vi "HO5_Generator#2.vi"(3 "?":bool, 4 "Delay (ms)":i16=500, 5 "Min":dbl=100.0, 6 "Max":dbl=500.0) -> (2 "Strip Chart":T2(graph))   [LabVIEW 2020]
panel:
  in  "Averaged Points":i16=5 min=1 max=1024 step=1
  out "Biggest/Smallest value":T1 {"Big time" format="%<%.3X>T"}
  out "Countdown (s)":dbl caption="Elapsed Time (s)"
  in  "Time Target (20)":dbl=20.0
  out "Current Overall average":dbl
  out "When slope is >0, than it's green.":bool
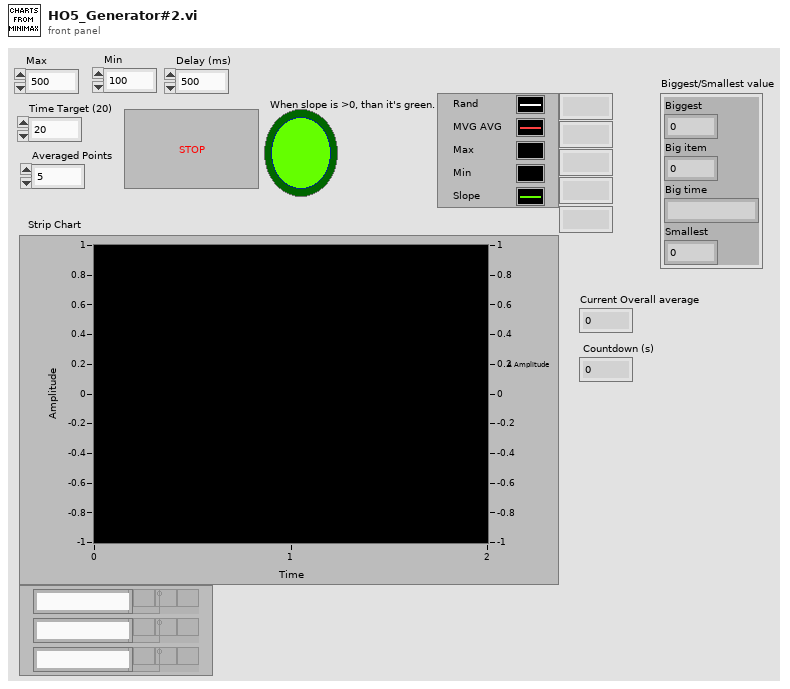
[diagram p1: front panel]
types:
  T1 = cluster{"Biggest":dbl, "Big item":i32, "Big time":timestamp, "Smallest":dbl}
  T2 = cluster{"Double":dbl, dbl, "Max":dbl, "Min":dbl, "Linear Slope":dbl}
  T3 = cluster{"Double":dbl, dbl, "Max":dbl, "Min":dbl, "Linear Slope":dbl}[]
  T4 = cluster{"Double":dbl, dbl, "Max":dbl, "Min":dbl, "Theta (degree)":dbl}
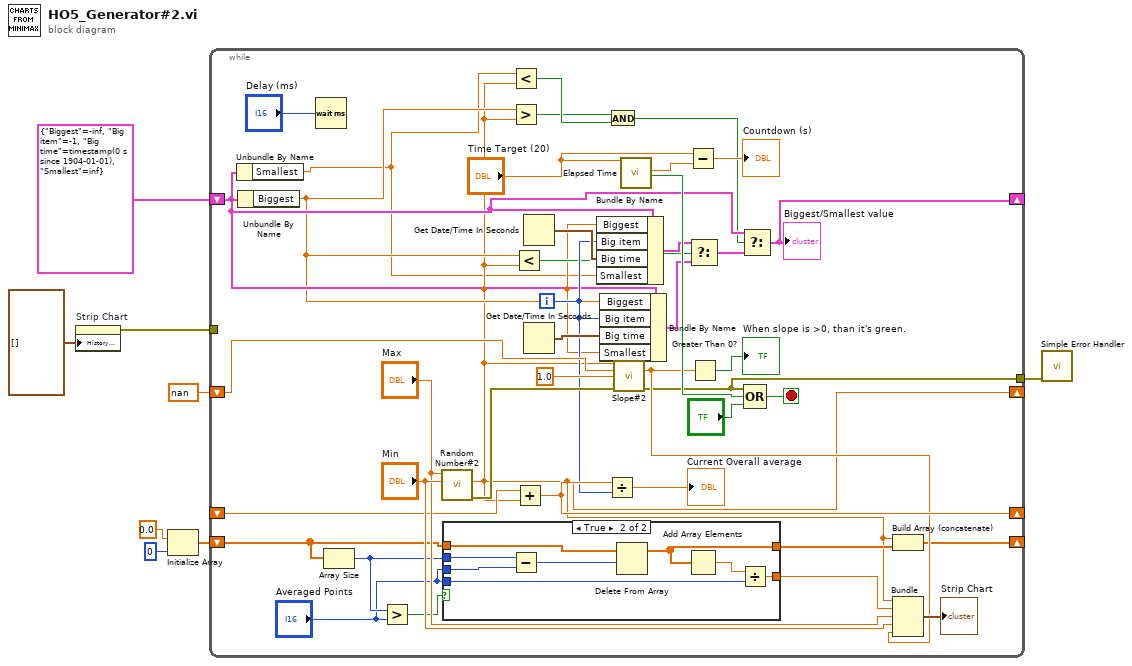
[diagram p0: block diagram]
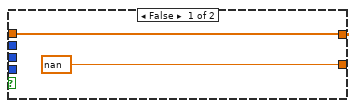
[diagram p2: hidden frame]
diagram:
  n1 = property on="Strip Chart" class="WFChart (strict)"("History Data"=T3 []) -> (error out=w8:errorcluster)  [unwired: 2 in, 1 out]
  n2 = Initialize Array(0.0 ("element"), 0 ("dimension size")) -> (w1:dbl[])
  n3 = while {
    tunnel: w8 -> [_]
    shift-right: [w42] -> _
    shift-left: _ -> [w43]
    tunnel: [w33] -> w6
    shift-right: [w12] -> _
    shift-left: nan -> [w32]
    shift-right: [w30] -> _
    shift-left: T1 {"Biggest"=-inf, "Big item"=-1, "Big time"=timestamp(0 s since 1904-01-01), "Smallest"=inf} -> [w26]
    shift-right: [w20] -> _
    shift-left: w1 -> [w18]
    i -> [w27]
    stop <- w41 stop-if-true
    n4 = Unbundle By Name(w26) -> ("Smallest"=w11:dbl)
    n5 = Unbundle By Name(w26) -> ("Biggest"=w13:dbl)
    n6 = Wait (ms)(milliseconds to wait="Delay (ms)") -> ()  [unwired: 1 out]
    n7 = Array Size(array=w18) -> (size(s)=w17:i32)
    n8 = Greater?(x=w17, y="Averaged Points") -> (0:w19:bool)
    n9 = call "Random Number#2.vi"("Maximum"="Max", "Minimum"="Min") -> ("Double"=w12:dbl, "error out"=w34:errorcluster)  [unwired: 4 in, 2 out]
    n10 = case shown="True" w19 {
      tunnel: w18 -> [w51 w59]
      tunnel: w17 -> [_ w57]
      tunnel: "Averaged Points" -> [_ w56]
      tunnel: "Averaged Points" -> [_ w55]
      tunnel: [nan w54] -> w15
      tunnel: [w51 w52] -> w14
      frame False {
      }
      frame True {
        n11 = Subtract(x=w57, y=w56) -> (x-y=w58:i32)
        n12 = Delete From Array(array=w59, length=w58) -> (array with subset deleted=w52:dbl[])  [unwired: 1 in, 1 out]
        n13 = Add Array Elements(numeric array=w52) -> (sum=w53:dbl)
        n14 = Divide(x=w53, y=w55) -> (x/y=w54:dbl)
      }
    }
    n15 = Less?(x=w11, y=w12) -> (x < y?=w25:bool)
    n16 = Greater?(x=w13, y=w12) -> (0:w22:bool)
    n17 = Less?(x=w13, y=w12) -> (x < y?=w21:bool)
    n18 = Add(x=w43, y=w12) -> (x+y=w42:dbl)
    n19 = Get Date/Time In Seconds() -> (seconds since 1Jan1904=w29:timestamp)
    n20 = Get Date/Time In Seconds() -> (seconds since 1Jan1904=w28:timestamp)
    n21 = Bundle By Name(cluster=w26, "Biggest"=w12, "Big item"=w27, "Big time"=w29, "Smallest"=w11) -> (w9:T1)
    n22 = Bundle By Name(cluster=w26, "Biggest"=w13, "Big item"=w27, "Big time"=w28, "Smallest"=w12) -> (w10:T1)
    n23 = Divide(x=w42, y=w27) -> (x/y=→"Current Overall average":dbl)
    n24 = And(x=w22, y=w25) -> (x .and. y?=w24:bool)
    n25 = call "Slope#2.vi"("Y2"=w12, "Y1"=w32, "X2 (1)"=1.0, "error in (no error)"=w34) -> ("Theta (degree)"=w35:dbl, "error out"=w33:errorcluster)  [unwired: 8 in, 2 out]
    n26 = call "Elapsed Time"("Time Target (s)"="Time Target (20)") -> ("Elapsed Time (s)"=w38:dbl, "Time has Elapsed"=w40:bool)  [unwired: 11 in, 6 out]
    n27 = Subtract(x="Time Target (20)", y=w38) -> (x-y=→"Countdown (s)":dbl)
    n28 = Select(t=w9, s=w21, f=w10) -> (s? t:f=w23:T1)
    n29 = Greater Than 0?(x=w35) -> (x > 0?=→"When slope is >0, than it's green.":bool)
    n30 = Select(t=w26, s=w24, f=w23) -> (s? t:f=w30:T1)
    "Biggest/Smallest value" <- w30
    n31 = Compound Arithmetic op=OR(w33, w40, "?") -> (w41:bool)
    n32 = Build Array (concatenate)(w12, w14) -> (w20:dbl[])
    n33 = Bundle("Double"=w12, w15, "Max"="Max", "Min"="Min", "Theta (degree)"=w35) -> (→"Strip Chart":T4)  [unwired: 1 in]
  }
  n34 = call <vilib>:"Simple Error Handler.vi"("error in (no error)"=w6) -> ()  [unwired: 4 in, 5 out]
